vi "TSM Relay PinTypeInfo.vi"() -> ()   [LabVIEW 2019]
doc: "LabVIEW Global used to store the Pin Type information (DUTPins vs. SystemPins) of all Pins declared in the user's Pin Map."
panel:
  in  "PinTypeInfo":T1
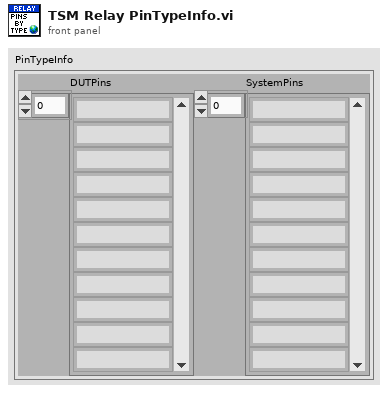
[diagram p1: front panel]
types:
  T1 = cluster{"DUTPins":string[], "SystemPins":string[]}
diagram:
